vi "Array Examples.vi"() -> ()   [LabVIEW 2020]
uses:
  <vilib>/sound2/lvsound2.llb/Sampling Mode.ctl
  <vilib>/sound2/lvsound2.llb/Sound Data Format.ctl
  <vilib>/sound2/lvsound2.llb/Sound Input Read (DBL).vi
panel:
  out "Channel 2 Data (Array)":dbl[](array[numeric])
  out "Channel 1 Data (Array)":dbl[](array[numeric])
  out "Sound Input - Waveform Array":waveform(dbl)[](array[waveform])
  in  "Device ID":u32
  out "Sound Input - Graph":waveform(dbl)[](graph)
  in  "Number of Samples/ch":i32=10000
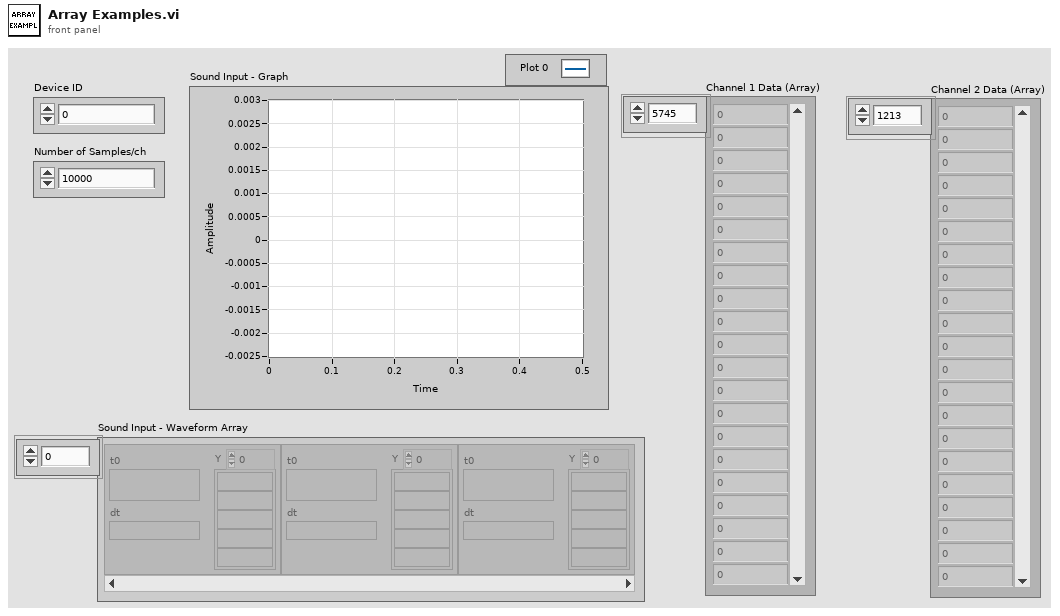
[diagram p1: front panel]
types:
  T1 = typedef "Sound Data Format.ctl" = cluster{"sample rate (S/s)":dbl, "number of channels":i32, "bits per sample":i32}
  T2 = typedef "Sampling Mode.ctl" = i32
  T3 = typedef "Sound Input Task ID.ctl" = u32
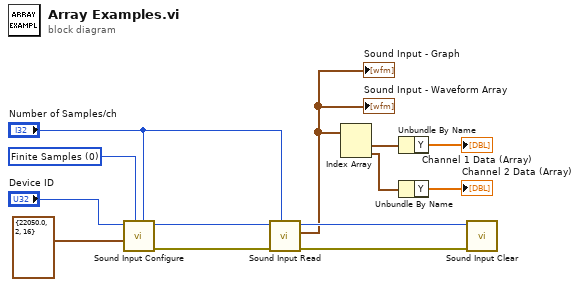
[diagram p0: block diagram]
diagram:
  w10 = T2 0 items=["Finite Samples", "Continuous Samples"] ("sample mode")
  n1 = call <vilib>:"Sound Input Configure.vi"("number of samples/ch"="Number of Samples/ch", "sample mode"=w10, "sound format"=T1 {"sample rate (S/s)"=22050.0, "number of channels"=2, "bits per sample"=16} ("Sound Format"), "device ID"="Device ID") -> ("error out"=w13:errorcluster, "task ID"=w11:T3)  [unwired: 6 in]
  n2 = call-poly <vilib>:"Sound Input Read.vi"("number of samples/ch"="Number of Samples/ch", "error in (no error)"=w13, "task ID"=w11) -> ("error out"=w8:errorcluster, "data"=w5:waveform(dbl)[], "task ID out"=w9:T3)  [unwired: 6 in]
  "Sound Input - Graph" <- w5
  "Sound Input - Waveform Array" <- w5
  n3 = Index Array(array=w5) -> (element #1=w3:waveform(dbl), element #2=w4:waveform(dbl))  [unwired: 2 in]
  n4 = Unbundle By Name(w3) -> ("Y"=→"Channel 1 Data (Array)":dbl[])
  n5 = Unbundle By Name(w4) -> ("Y"=→"Channel 2 Data (Array)":dbl[])
  n6 = call <vilib>:"Sound Input Clear.vi"("error in (no error)"=w8, "task ID"=w9) -> ()  [unwired: 9 in, 1 out]
